vi "主程序面板.vi"() -> ()   [LabVIEW 2018]
panel:
  in  "跳转按钮":bool
  in  "确定":bool
  in  "程序停止":bool
  in  "室内火焰分割算法":u16(ring) items=["请选择所需算法", "Canny算法分割", "Otsu算法分割"]
  in  "室外火焰分割算法":u16(ring) items=["请选择所需算法", "默认系数进行阈值分割", "单幅图像系数分割"]
  in  "室内外火焰分割算法":u16(ring) items=["请选择所需算法", "手动设定阈值分割", "单幅图像阈值分割"]
  # "火焰图像处理算法选择"
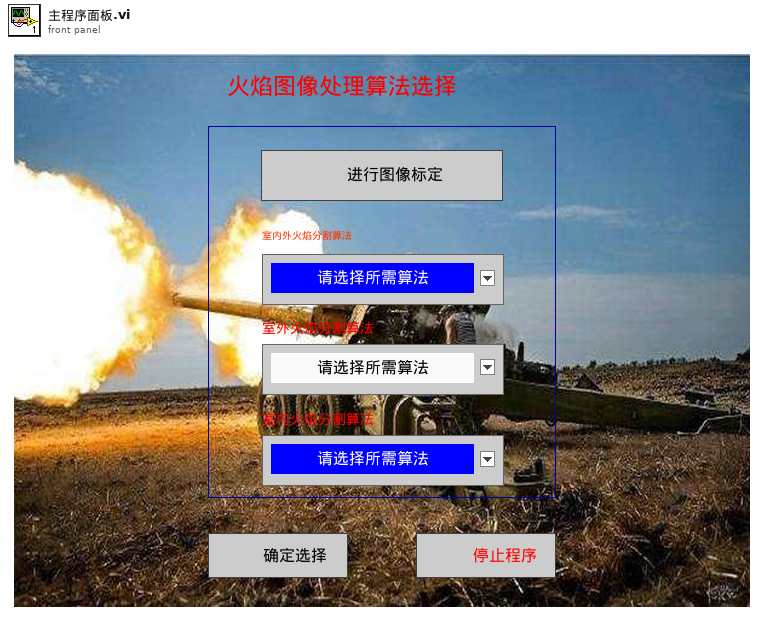
[diagram p1: front panel]
types:
  T1 = enum32{"Invalid", "Standard", "Closed", "Hidden", "Minimized", "Maximized"}
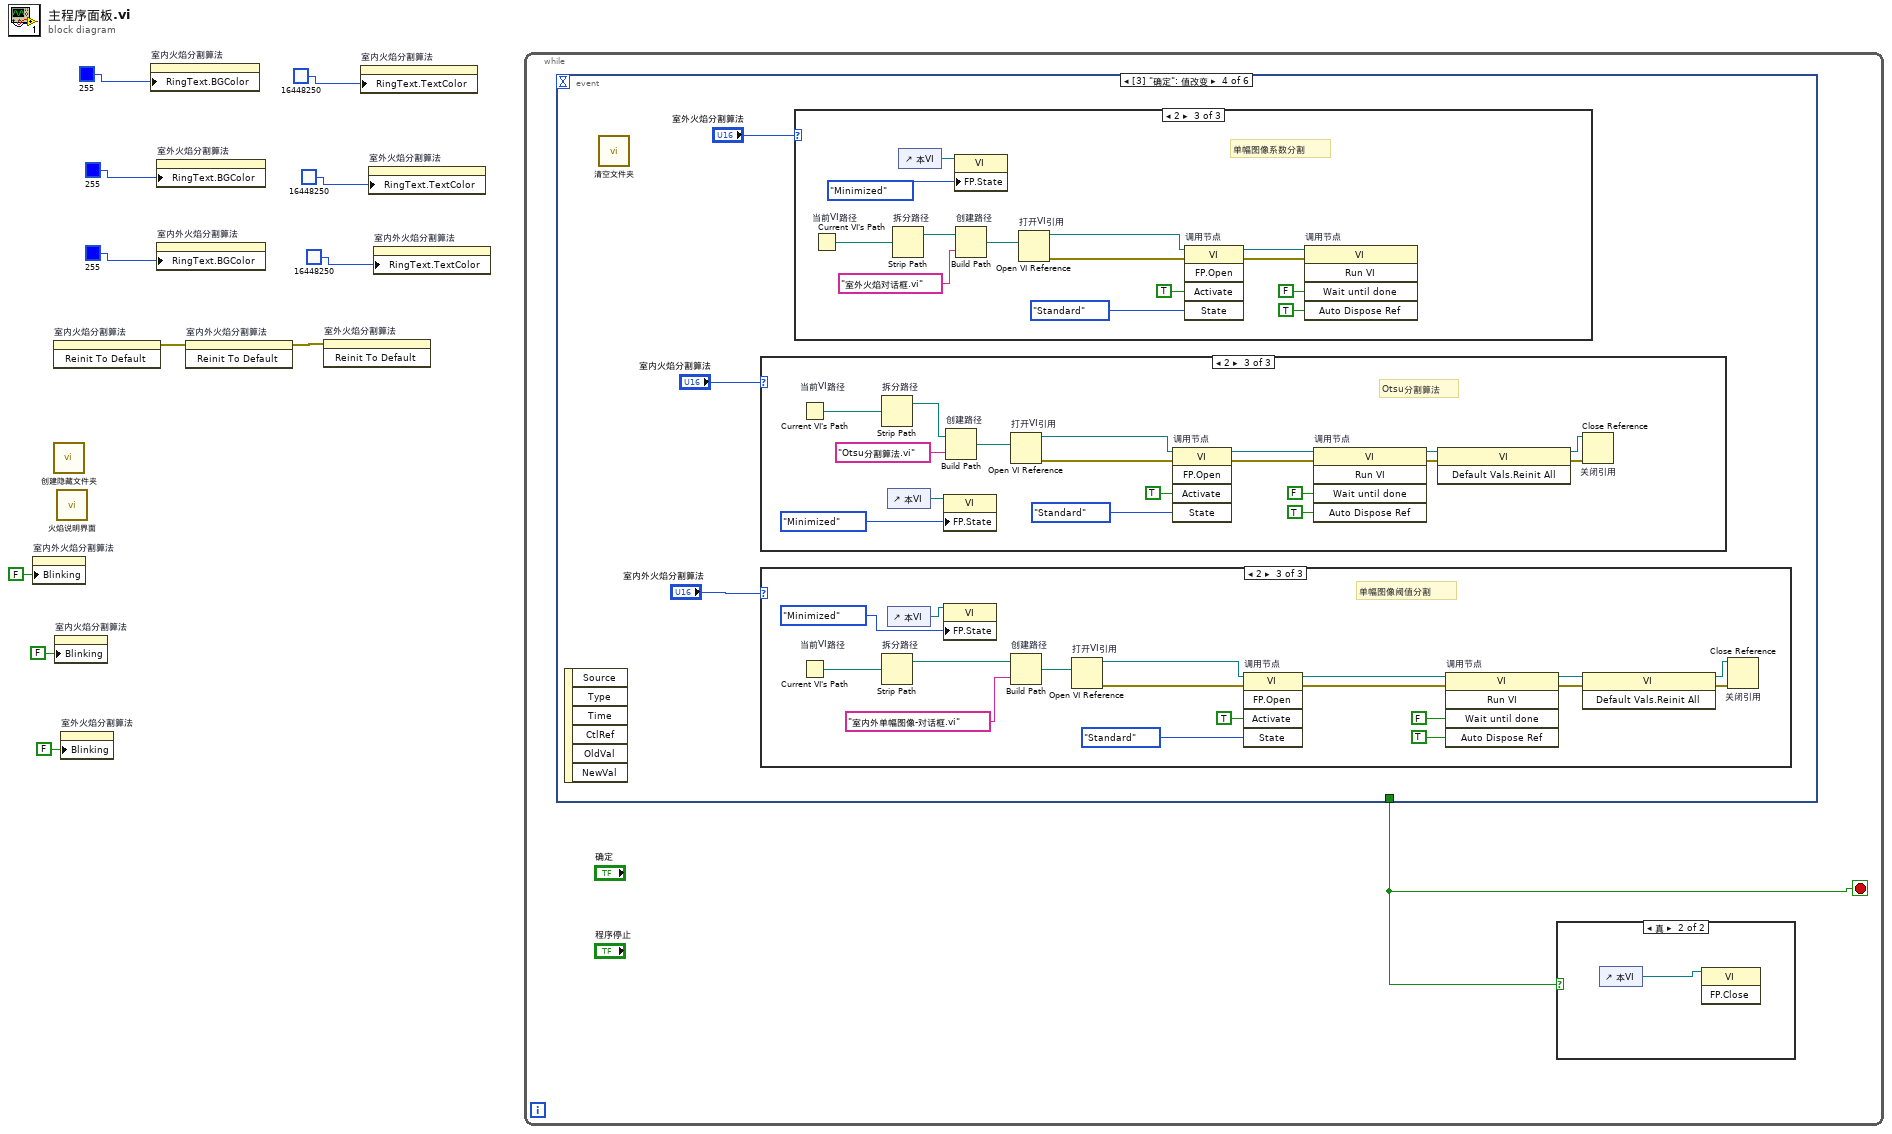
[diagram p0: block diagram]
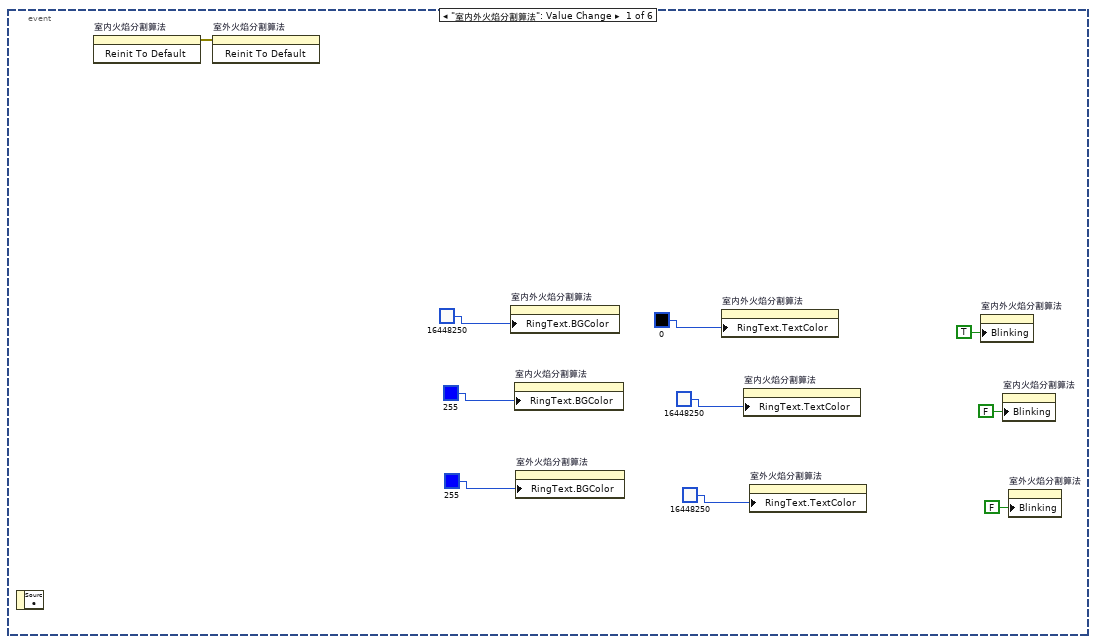
[diagram p3: hidden frame]
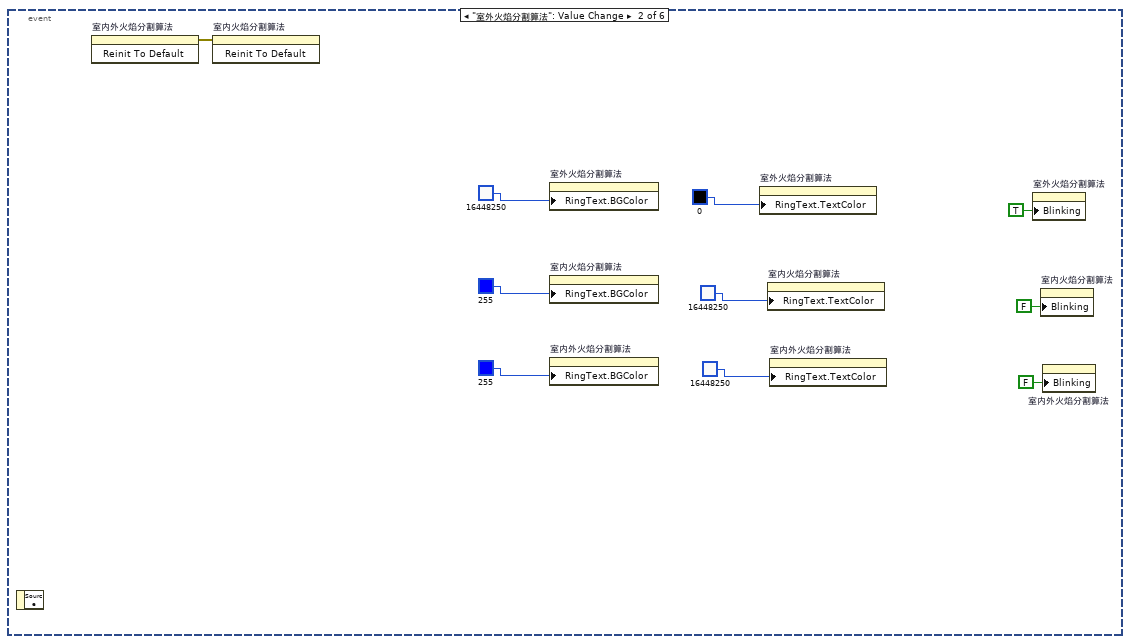
[diagram p4: hidden frame]
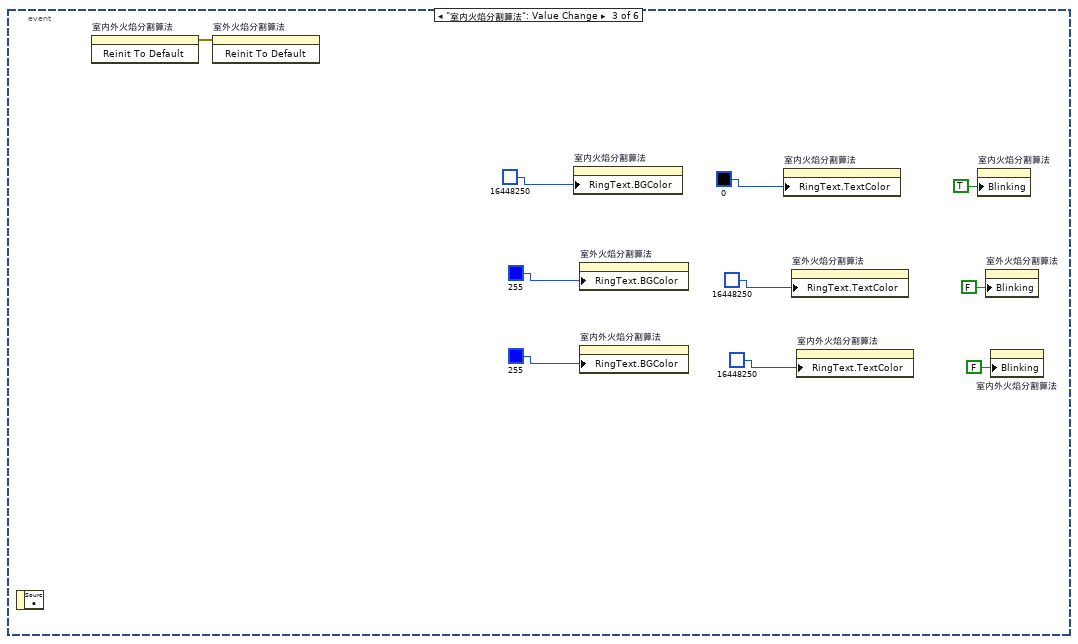
[diagram p5: hidden frame]
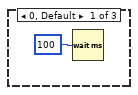
[diagram p6: hidden frame]
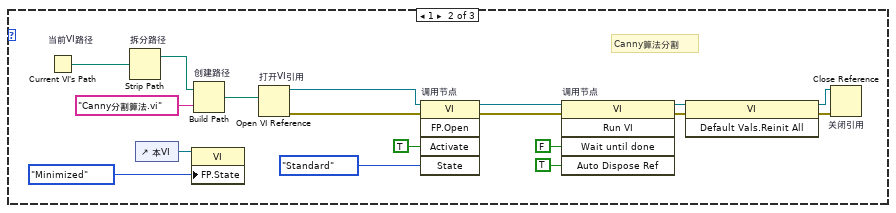
[diagram p7: hidden frame]
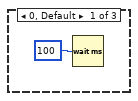
[diagram p8: hidden frame]
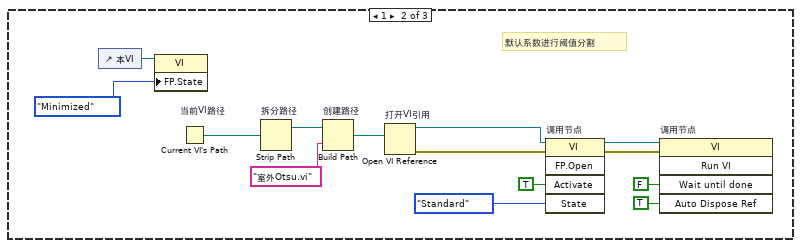
[diagram p9: hidden frame]
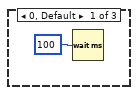
[diagram p10: hidden frame]
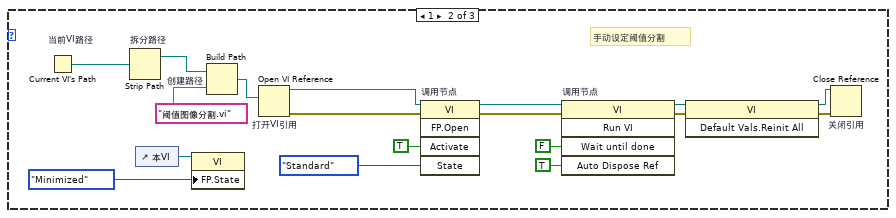
[diagram p11: hidden frame]
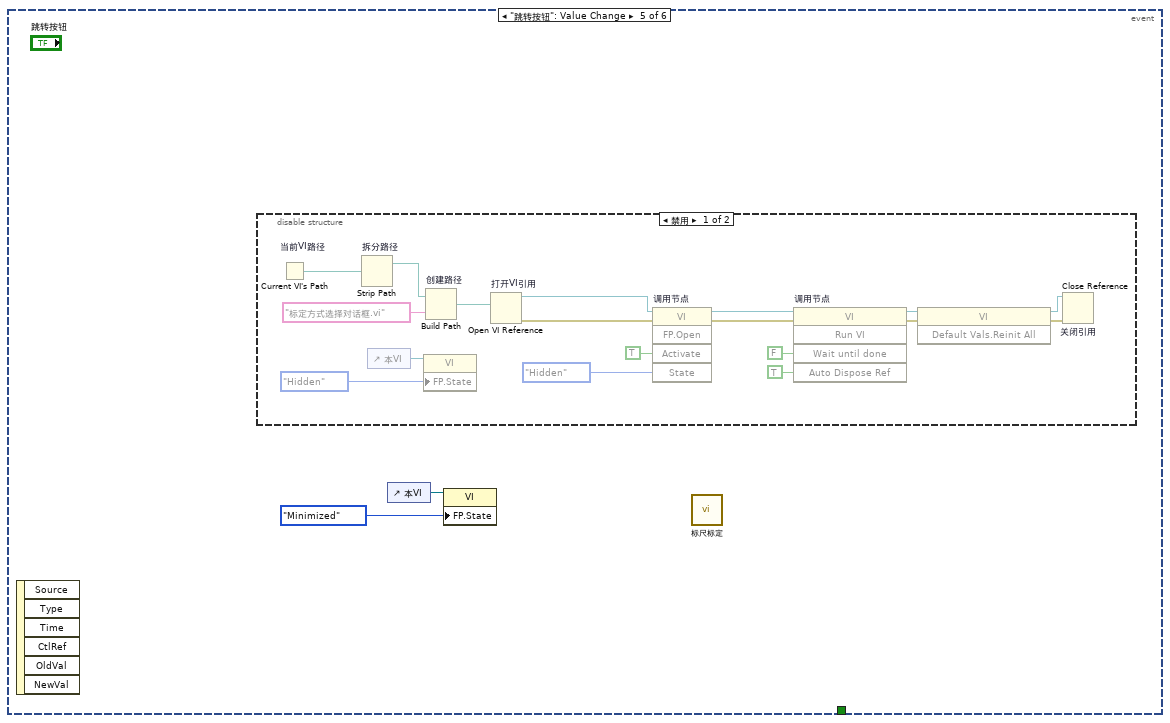
[diagram p12: hidden frame]
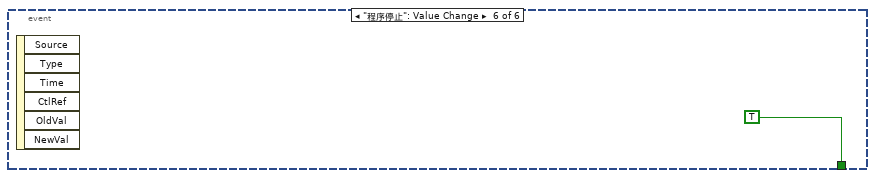
[diagram p14: hidden frame]
diagram:
  n1 = property on="室内外火焰分割算法" class="Ring (严格)"("Blinking"=FALSE ("闪烁")) -> ()  [unwired: 2 in, 2 out]
  n2 = invoke on="室内火焰分割算法" class="Ring (严格)" method="Reinit To Default"() -> (error out=w4:errorcluster)  [unwired: 3 in, 2 out]
  n3 = call "创建隐藏文件夹.vi"() -> ()  [unwired: 12 in]
  n4 = property on="室内火焰分割算法" class="Ring (严格)"("Blinking"=FALSE ("闪烁")) -> ()  [unwired: 2 in, 2 out]
  n5 = call "火焰说明界面.vi"() -> ()  [unwired: 12 in]
  n6 = property on="室外火焰分割算法" class="Ring (严格)"("Blinking"=FALSE ("闪烁")) -> ()  [unwired: 2 in, 2 out]
  n7 = property on="室内火焰分割算法" class="Ring (严格)"("RingText.BGColor"=u32 255) -> ()  [unwired: 2 in, 2 out]
  n8 = property on="室外火焰分割算法" class="Ring (严格)"("RingText.BGColor"=u32 255) -> ()  [unwired: 2 in, 2 out]
  n9 = property on="室内外火焰分割算法" class="Ring (严格)"("RingText.BGColor"=u32 255) -> ()  [unwired: 2 in, 2 out]
  n10 = invoke on="室内外火焰分割算法" class="Ring (严格)" method="Reinit To Default"(error in=w4) -> (error out=w5:errorcluster)  [unwired: 2 in, 2 out]
  n11 = invoke on="室外火焰分割算法" class="Ring (严格)" method="Reinit To Default"(error in=w5) -> ()  [unwired: 2 in, 3 out]
  n12 = property on="室内火焰分割算法" class="Ring (严格)"("RingText.TextColor"=u32 16448250) -> ()  [unwired: 2 in, 2 out]
  n13 = property on="室外火焰分割算法" class="Ring (严格)"("RingText.TextColor"=u32 16448250) -> ()  [unwired: 2 in, 2 out]
  n14 = property on="室内外火焰分割算法" class="Ring (严格)"("RingText.TextColor"=u32 16448250) -> ()  [unwired: 2 in, 2 out]
  n15 = while {
    stop <- w12 stop-if-true
    n16 = event shown="[3] \"确定\": 值改变" {
      selector: _ -> [_ _ _ _ _ _]
      dyn-events: _ -> [_ _ _ _ _ _]
      timeout: _ -> [_ _ _ _ _ _]
      tunnel: [_ _ _ _ _ TRUE] -> w12
      event "室内外火焰分割算法": Value Change {
        n17 = event-data() -> ()  [unwired: 1 in, 1 out]
        n18 = invoke on="室内火焰分割算法" class="Ring (严格)" method="Reinit To Default"() -> (error out=w23:errorcluster)  [unwired: 3 in, 2 out]
        n19 = invoke on="室外火焰分割算法" class="Ring (严格)" method="Reinit To Default"(error in=w23) -> ()  [unwired: 2 in, 3 out]
        n20 = property on="室内外火焰分割算法" class="Ring (严格)"("RingText.BGColor"=u32 16448250) -> ()  [unwired: 2 in, 2 out]
        n21 = property on="室内火焰分割算法" class="Ring (严格)"("RingText.BGColor"=u32 255) -> ()  [unwired: 2 in, 2 out]
        n22 = property on="室外火焰分割算法" class="Ring (严格)"("RingText.BGColor"=u32 255) -> ()  [unwired: 2 in, 2 out]
        n23 = property on="室内外火焰分割算法" class="Ring (严格)"("RingText.TextColor"=u32 0) -> ()  [unwired: 2 in, 2 out]
        n24 = property on="室内火焰分割算法" class="Ring (严格)"("RingText.TextColor"=u32 16448250) -> ()  [unwired: 2 in, 2 out]
        n25 = property on="室外火焰分割算法" class="Ring (严格)"("RingText.TextColor"=u32 16448250) -> ()  [unwired: 2 in, 2 out]
        n26 = property on="室内外火焰分割算法" class="Ring (严格)"("Blinking"=TRUE ("闪烁")) -> ()  [unwired: 2 in, 2 out]
        n27 = property on="室内火焰分割算法" class="Ring (严格)"("Blinking"=FALSE ("闪烁")) -> ()  [unwired: 2 in, 2 out]
        n28 = property on="室外火焰分割算法" class="Ring (严格)"("Blinking"=FALSE ("闪烁")) -> ()  [unwired: 2 in, 2 out]
      }
      event "室外火焰分割算法": Value Change {
        n29 = event-data() -> ()  [unwired: 1 in, 1 out]
        n30 = invoke on="室内外火焰分割算法" class="Ring (严格)" method="Reinit To Default"() -> (error out=w33:errorcluster)  [unwired: 3 in, 2 out]
        n31 = invoke on="室内火焰分割算法" class="Ring (严格)" method="Reinit To Default"(error in=w33) -> ()  [unwired: 2 in, 3 out]
        n32 = property on="室外火焰分割算法" class="Ring (严格)"("RingText.BGColor"=u32 16448250) -> ()  [unwired: 2 in, 2 out]
        n33 = property on="室内火焰分割算法" class="Ring (严格)"("RingText.BGColor"=u32 255) -> ()  [unwired: 2 in, 2 out]
        n34 = property on="室内外火焰分割算法" class="Ring (严格)"("RingText.BGColor"=u32 255) -> ()  [unwired: 2 in, 2 out]
        n35 = property on="室外火焰分割算法" class="Ring (严格)"("RingText.TextColor"=u32 0) -> ()  [unwired: 2 in, 2 out]
        n36 = property on="室内火焰分割算法" class="Ring (严格)"("RingText.TextColor"=u32 16448250) -> ()  [unwired: 2 in, 2 out]
        n37 = property on="室内外火焰分割算法" class="Ring (严格)"("RingText.TextColor"=u32 16448250) -> ()  [unwired: 2 in, 2 out]
        n38 = property on="室外火焰分割算法" class="Ring (严格)"("Blinking"=TRUE ("闪烁")) -> ()  [unwired: 2 in, 2 out]
        n39 = property on="室内火焰分割算法" class="Ring (严格)"("Blinking"=FALSE ("闪烁")) -> ()  [unwired: 2 in, 2 out]
        n40 = property on="室内外火焰分割算法" class="Ring (严格)"("Blinking"=FALSE ("闪烁")) -> ()  [unwired: 2 in, 2 out]
      }
      event "室内火焰分割算法": Value Change {
        n41 = event-data() -> ()  [unwired: 1 in, 1 out]
        n42 = invoke on="室内外火焰分割算法" class="Ring (严格)" method="Reinit To Default"() -> (error out=w43:errorcluster)  [unwired: 3 in, 2 out]
        n43 = invoke on="室外火焰分割算法" class="Ring (严格)" method="Reinit To Default"(error in=w43) -> ()  [unwired: 2 in, 3 out]
        n44 = property on="室内火焰分割算法" class="Ring (严格)"("RingText.BGColor"=u32 16448250) -> ()  [unwired: 2 in, 2 out]
        n45 = property on="室外火焰分割算法" class="Ring (严格)"("RingText.BGColor"=u32 255) -> ()  [unwired: 2 in, 2 out]
        n46 = property on="室内外火焰分割算法" class="Ring (严格)"("RingText.BGColor"=u32 255) -> ()  [unwired: 2 in, 2 out]
        n47 = property on="室内火焰分割算法" class="Ring (严格)"("RingText.TextColor"=u32 0) -> ()  [unwired: 2 in, 2 out]
        n48 = property on="室外火焰分割算法" class="Ring (严格)"("RingText.TextColor"=u32 16448250) -> ()  [unwired: 2 in, 2 out]
        n49 = property on="室内外火焰分割算法" class="Ring (严格)"("RingText.TextColor"=u32 16448250) -> ()  [unwired: 2 in, 2 out]
        n50 = property on="室内火焰分割算法" class="Ring (严格)"("Blinking"=TRUE ("闪烁")) -> ()  [unwired: 2 in, 2 out]
        n51 = property on="室外火焰分割算法" class="Ring (严格)"("Blinking"=FALSE ("闪烁")) -> ()  [unwired: 2 in, 2 out]
        n52 = property on="室内外火焰分割算法" class="Ring (严格)"("Blinking"=FALSE ("闪烁")) -> ()  [unwired: 2 in, 2 out]
      }
      event "确定": Value Change {
        n53 = event-data() -> ()  [unwired: 1 in, 6 out]
        n54 = call "清空文件夹.vi"() -> ()  [unwired: 12 in]
        n55 = case shown="2" "室内火焰分割算法" {
          frame 0, Default {
            n56 = Wait (ms)(milliseconds to wait=u32 100 ("等待时间（毫秒）")) -> ()  [unwired: 1 out]
          }
          frame 1 {
            # "Canny算法分割"
            n57 = Current VI's Path "当前VI路径"() -> (path=w61:path)
            n58 = Strip Path "拆分路径"(path=w61) -> (stripped path=w65:path)  [unwired: 1 out]
            n59 = control-ref of="本VI"() -> (w49:refnum<vi>)
            n60 = property class="VI"(reference=w49, "FP.State"=T1."Minimized" ("前面板窗口:状态")) -> ()  [unwired: 1 in, 2 out]
            n61 = Build Path "创建路径"(base path=w65, name or relative path="Canny分割算法.vi" ("名称或相对路径")) -> (appended path=w62:path)
            n62 = Open VI Reference "打开VI引用"(vi path=w62) -> (vi reference=w59:refnum<vi>, error out=w58:errorcluster)  [unwired: 5 in]
            n63 = invoke on="调用节点" class="VI" method="FP.Open"(reference=w59, error in=w58, "Activate"=TRUE ("激活？"), "State"=T1."Standard" ("状态")) -> (reference out=w57:refnum<vi>, error out=w56:errorcluster)  [unwired: 1 in, 3 out]
            n64 = invoke on="调用节点" class="VI" method="Run VI"(reference=w57, error in=w56, "Wait until done"=FALSE ("结束前等待"), "Auto Dispose Ref"=TRUE ("自动销毁引用")) -> (reference out=w53:refnum<vi>, error out=w52:errorcluster)  [unwired: 1 in, 3 out]
            n65 = invoke class="VI" method="Default Vals.Reinit All"(reference=w53, error in=w52) -> (reference out=w51:refnum<vi>, error out=w50:errorcluster)  [unwired: 1 in, 1 out]
            n66 = Close Reference "关闭引用"(reference=w51, error in (no error)=w50) -> ()  [unwired: 1 out]
          }
          frame 2 {
            # "Otsu分割算法"
            n67 = Current VI's Path "当前VI路径"() -> (path=w78:path)
            n68 = Strip Path "拆分路径"(path=w78) -> (stripped path=w83:path)  [unwired: 1 out]
            n69 = control-ref of="本VI"() -> (w67:refnum<vi>)
            n70 = property class="VI"(reference=w67, "FP.State"=T1."Minimized" ("前面板窗口:状态")) -> ()  [unwired: 1 in, 2 out]
            n71 = Build Path "创建路径"(base path=w83, name or relative path="Otsu分割算法.vi" ("名称或相对路径")) -> (appended path=w79:path)
            n72 = Open VI Reference "打开VI引用"(vi path=w79) -> (vi reference=w76:refnum<vi>, error out=w75:errorcluster)  [unwired: 5 in]
            n73 = invoke on="调用节点" class="VI" method="FP.Open"(reference=w76, error in=w75, "Activate"=TRUE ("激活？"), "State"=T1."Standard" ("状态")) -> (reference out=w74:refnum<vi>, error out=w73:errorcluster)  [unwired: 1 in, 3 out]
            n74 = invoke on="调用节点" class="VI" method="Run VI"(reference=w74, error in=w73, "Wait until done"=FALSE ("结束前等待"), "Auto Dispose Ref"=TRUE ("自动销毁引用")) -> (reference out=w71:refnum<vi>, error out=w69:errorcluster)  [unwired: 1 in, 3 out]
            n75 = invoke class="VI" method="Default Vals.Reinit All"(reference=w71, error in=w69) -> (reference out=w70:refnum<vi>, error out=w68:errorcluster)  [unwired: 1 in, 1 out]
            n76 = Close Reference "关闭引用"(reference=w70, error in (no error)=w68) -> ()  [unwired: 1 out]
          }
        }
        n77 = case shown="2" "室内外火焰分割算法" {
          frame 0, Default {
            n78 = Wait (ms)(milliseconds to wait=u32 100 ("等待时间（毫秒）")) -> ()  [unwired: 1 out]
          }
          frame 1 {
            # "手动设定阈值分割"
            n79 = Current VI's Path "当前VI路径"() -> (path=w126:path)
            n80 = Strip Path "拆分路径"(path=w126) -> (stripped path=w131:path)  [unwired: 1 out]
            n81 = control-ref of="本VI"() -> (w115:refnum<vi>)
            n82 = property class="VI"(reference=w115, "FP.State"=T1."Minimized" ("前面板窗口:状态")) -> ()  [unwired: 1 in, 2 out]
            n83 = Build Path "创建路径"(base path=w131, name or relative path="阈值图像分割.vi" ("名称或相对路径")) -> (appended path=w127:path)
            n84 = Open VI Reference "打开VI引用"(vi path=w127) -> (vi reference=w124:refnum<vi>, error out=w123:errorcluster)  [unwired: 5 in]
            n85 = invoke on="调用节点" class="VI" method="FP.Open"(reference=w124, error in=w123, "Activate"=TRUE ("激活？"), "State"=T1."Standard" ("状态")) -> (reference out=w122:refnum<vi>, error out=w121:errorcluster)  [unwired: 1 in, 3 out]
            n86 = invoke on="调用节点" class="VI" method="Run VI"(reference=w122, error in=w121, "Wait until done"=FALSE ("结束前等待"), "Auto Dispose Ref"=TRUE ("自动销毁引用")) -> (reference out=w119:refnum<vi>, error out=w117:errorcluster)  [unwired: 1 in, 3 out]
            n87 = invoke class="VI" method="Default Vals.Reinit All"(reference=w119, error in=w117) -> (reference out=w118:refnum<vi>, error out=w116:errorcluster)  [unwired: 1 in, 1 out]
            n88 = Close Reference "关闭引用"(reference=w118, error in (no error)=w116) -> ()  [unwired: 1 out]
          }
          frame 2 {
            # "单幅图像阈值分割"
            n89 = Current VI's Path "当前VI路径"() -> (path=w145:path)
            n90 = Strip Path "拆分路径"(path=w145) -> (stripped path=w149:path)  [unwired: 1 out]
            n91 = control-ref of="本VI"() -> (w133:refnum<vi>)
            n92 = property class="VI"(reference=w133, "FP.State"=T1."Minimized" ("前面板窗口:状态")) -> ()  [unwired: 1 in, 2 out]
            n93 = Build Path "创建路径"(base path=w149, name or relative path="室内外单幅图像-对话框.vi" ("名称或相对路径")) -> (appended path=w146:path)
            n94 = Open VI Reference "打开VI引用"(vi path=w146) -> (vi reference=w143:refnum<vi>, error out=w142:errorcluster)  [unwired: 5 in]
            n95 = invoke on="调用节点" class="VI" method="FP.Open"(reference=w143, error in=w142, "Activate"=TRUE ("激活？"), "State"=T1."Standard" ("状态")) -> (reference out=w141:refnum<vi>, error out=w140:errorcluster)  [unwired: 1 in, 3 out]
            n96 = invoke on="调用节点" class="VI" method="Run VI"(reference=w141, error in=w140, "Wait until done"=FALSE ("结束前等待"), "Auto Dispose Ref"=TRUE ("自动销毁引用")) -> (reference out=w137:refnum<vi>, error out=w136:errorcluster)  [unwired: 1 in, 3 out]
            n97 = invoke class="VI" method="Default Vals.Reinit All"(reference=w137, error in=w136) -> (reference out=w135:refnum<vi>, error out=w134:errorcluster)  [unwired: 1 in, 1 out]
            n98 = Close Reference "关闭引用"(reference=w135, error in (no error)=w134) -> ()  [unwired: 1 out]
          }
        }
        n99 = case shown="2" "室外火焰分割算法" {
          frame 0, Default {
            n100 = Wait (ms)(milliseconds to wait=u32 100 ("等待时间（毫秒）")) -> ()  [unwired: 1 out]
          }
          frame 1 {
            # "默认系数进行阈值分割"
            n101 = control-ref of="本VI"() -> (w86:refnum<vi>)
            n102 = property class="VI"(reference=w86, "FP.State"=T1."Minimized" ("前面板窗口:状态")) -> ()  [unwired: 1 in, 2 out]
            n103 = Current VI's Path "当前VI路径"() -> (path=w94:path)
            n104 = Strip Path "拆分路径"(path=w94) -> (stripped path=w98:path)  [unwired: 1 out]
            n105 = Build Path "创建路径"(base path=w98, name or relative path="室外Otsu.vi" ("名称或相对路径")) -> (appended path=w95:path)
            n106 = Open VI Reference "打开VI引用"(vi path=w95) -> (vi reference=w92:refnum<vi>, error out=w91:errorcluster)  [unwired: 5 in]
            n107 = invoke on="调用节点" class="VI" method="FP.Open"(reference=w92, error in=w91, "Activate"=TRUE ("激活？"), "State"=T1."Standard" ("状态")) -> (reference out=w90:refnum<vi>, error out=w89:errorcluster)  [unwired: 1 in, 3 out]
            n108 = invoke on="调用节点" class="VI" method="Run VI"(reference=w90, error in=w89, "Wait until done"=FALSE ("结束前等待"), "Auto Dispose Ref"=TRUE ("自动销毁引用")) -> ()  [unwired: 1 in, 5 out]
          }
          frame 2 {
            # "单幅图像系数分割"
            n109 = Current VI's Path "当前VI路径"() -> (path=w108:path)
            n110 = Strip Path "拆分路径"(path=w108) -> (stripped path=w106:path)  [unwired: 1 out]
            n111 = control-ref of="本VI"() -> (w99:refnum<vi>)
            n112 = property class="VI"(reference=w99, "FP.State"=T1."Minimized" ("前面板窗口:状态")) -> ()  [unwired: 1 in, 2 out]
            n113 = Build Path "创建路径"(base path=w106, name or relative path="室外火焰对话框.vi" ("名称或相对路径")) -> (appended path=w107:path)
            n114 = Open VI Reference "打开VI引用"(vi path=w107) -> (vi reference=w109:refnum<vi>, error out=w110:errorcluster)  [unwired: 5 in]
            n115 = invoke on="调用节点" class="VI" method="FP.Open"(reference=w109, error in=w110, "Activate"=TRUE ("激活？"), "State"=T1."Standard" ("状态")) -> (reference out=w111:refnum<vi>, error out=w112:errorcluster)  [unwired: 1 in, 3 out]
            n116 = invoke on="调用节点" class="VI" method="Run VI"(reference=w111, error in=w112, "Wait until done"=FALSE ("结束前等待"), "Auto Dispose Ref"=TRUE ("自动销毁引用")) -> ()  [unwired: 1 in, 5 out]
          }
        }
      }
      event "跳转按钮": Value Change {
        n117 = event-data() -> ()  [unwired: 1 in, 6 out]
        n118 = disable-structure shown="禁用" {
          frame Disabled {
            n119 = Current VI's Path "当前VI路径"() -> (path=w164:path)
            n120 = Strip Path "拆分路径"(path=w164) -> (stripped path=w169:path)  [unwired: 1 out]
            n121 = control-ref of="本VI"() -> (w153:refnum<vi>)
            n122 = property class="VI"(reference=w153, "FP.State"=T1."Hidden" ("前面板窗口:状态")) -> ()  [unwired: 1 in, 2 out]
            n123 = Build Path "创建路径"(base path=w169, name or relative path="标定方式选择对话框.vi" ("名称或相对路径")) -> (appended path=w165:path)
            n124 = Open VI Reference "打开VI引用"(vi path=w165) -> (vi reference=w162:refnum<vi>, error out=w161:errorcluster)  [unwired: 5 in]
            n125 = invoke on="调用节点" class="VI" method="FP.Open"(reference=w162, error in=w161, "Activate"=TRUE ("激活？"), "State"=T1."Hidden" ("状态")) -> (reference out=w160:refnum<vi>, error out=w159:errorcluster)  [unwired: 1 in, 3 out]
            n126 = invoke on="调用节点" class="VI" method="Run VI"(reference=w160, error in=w159, "Wait until done"=FALSE ("结束前等待"), "Auto Dispose Ref"=TRUE ("自动销毁引用")) -> (reference out=w157:refnum<vi>, error out=w155:errorcluster)  [unwired: 1 in, 3 out]
            n127 = invoke class="VI" method="Default Vals.Reinit All"(reference=w157, error in=w155) -> (reference out=w156:refnum<vi>, error out=w154:errorcluster)  [unwired: 1 in, 1 out]
            n128 = Close Reference "关闭引用"(reference=w156, error in (no error)=w154) -> ()  [unwired: 1 out]
          }
          frame Enabled {
          }
        }
        n129 = control-ref of="本VI"() -> (w150:refnum<vi>)
        n130 = property class="VI"(reference=w150, "FP.State"=T1."Minimized" ("前面板窗口:状态")) -> ()  [unwired: 1 in, 2 out]
        n131 = call "标尺标定.vi"() -> ()  [unwired: 12 in]
      }
      event "程序停止": Value Change {
        n132 = event-data() -> ()  [unwired: 1 in, 6 out]
      }
    }
    n133 = case shown="真" w12 {
      frame False {
      }
      frame True {
        n134 = control-ref of="本VI"() -> (w13:refnum<vi>)
        n135 = invoke class="VI" method="FP.Close"(reference=w13) -> ()  [unwired: 2 in, 3 out]
      }
    }
  }
